vi "Spindle_load_RT_truncated (SubVI).vi"(9 "?":T1, 10 "concatenated string 4":string, 11 "String":string) -> (0 "error out":errorcluster, 1 "content 4":string, 2 "content1 2":string, 3 "output cluster":T1, 4 "empty? 2":bool, 5 "concatenated string":string, 6 "load":string, 7 "concatenated string 2":string)   [LabVIEW 2017]
uses:
  MT_connect_data.ctl
  <vilib>/regexp/Match Regular Expression.xnode
  <vilib>/addons/internet/NI_InternetTK_Core_VIs.lvlib
panel:
  out "Position A 2":string
  out "content 7":string
  out "content 6":string
  out "after match":string
  out "Z_position":string
  out "X_position":string
  out "Y_poistion":string
  out "concatenated string 6":string
  out "content 3":string
  out "Position B":string
  out "content 2":string
  out "concatenated string 5":string
  out "Position A":string
  out "Avail":string
  out "Tool_ID":string
  out "Program_name":string
  out "Controller_Mode":string
  out "Line_code":string
  out "program_status":string
  out "Block":string
  out "feeover":string
  out "Speedover":string
  out "path feedrate":string
  out "content":string
  out "error out 2":errorcluster
  out "spindle speed":string
  out "content 5":string
  out "empty? 3":bool
  out "after match 3":string
  out "content1 3":string
  out "concatenated string 3":string
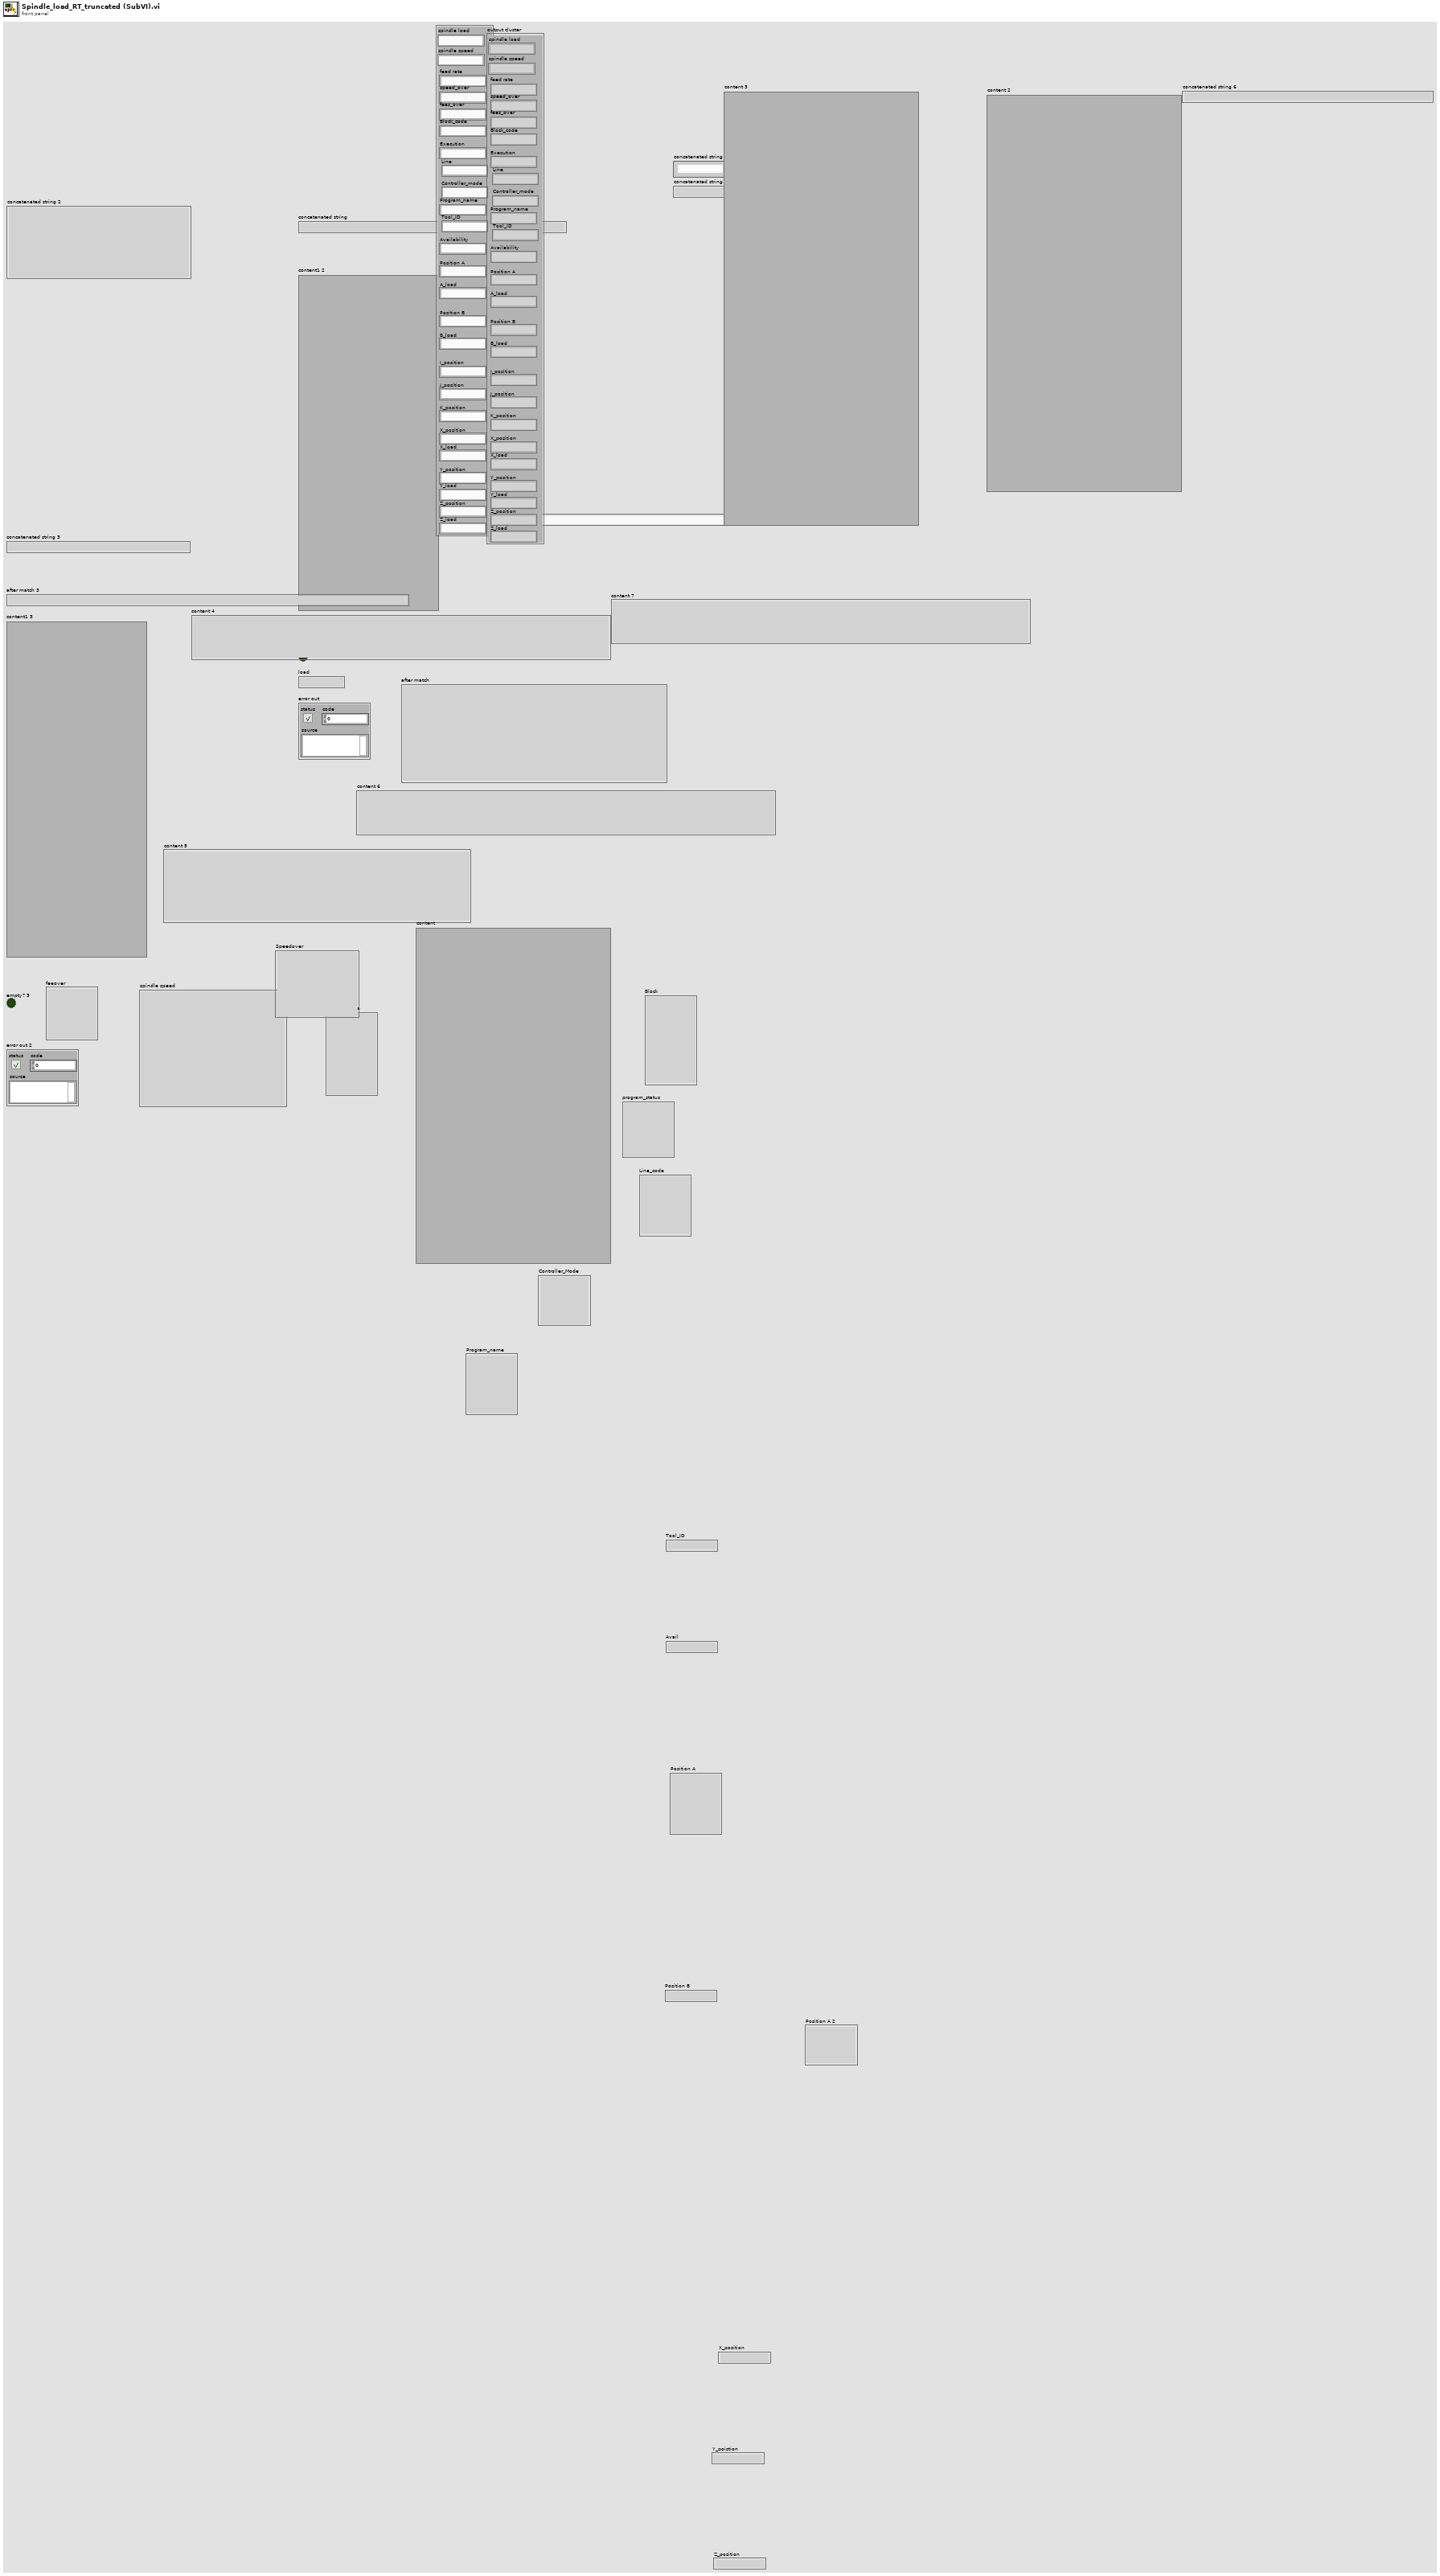
[diagram p1: front panel]
types:
  T1 = typedef "MT_connect_data.ctl" = cluster{"spindle load ":string, "spindle speed ":string, "feed rate":string, "speed_over":string, "fees_over":string, "Block_code":string, "Execution":string, "Line":string, "Controller_mode":string, "Program_name":string, "Tool_ID":string, "Availability":string, "Position A":string, "A_load":string, "Position B":string, "B_load":string, "I_position":string, "J_position":string, "K_position":string, "X_position":string, "X_load":string, "Y_position":string, "Y_load":string, "Z_position":string, "Z_load":string}
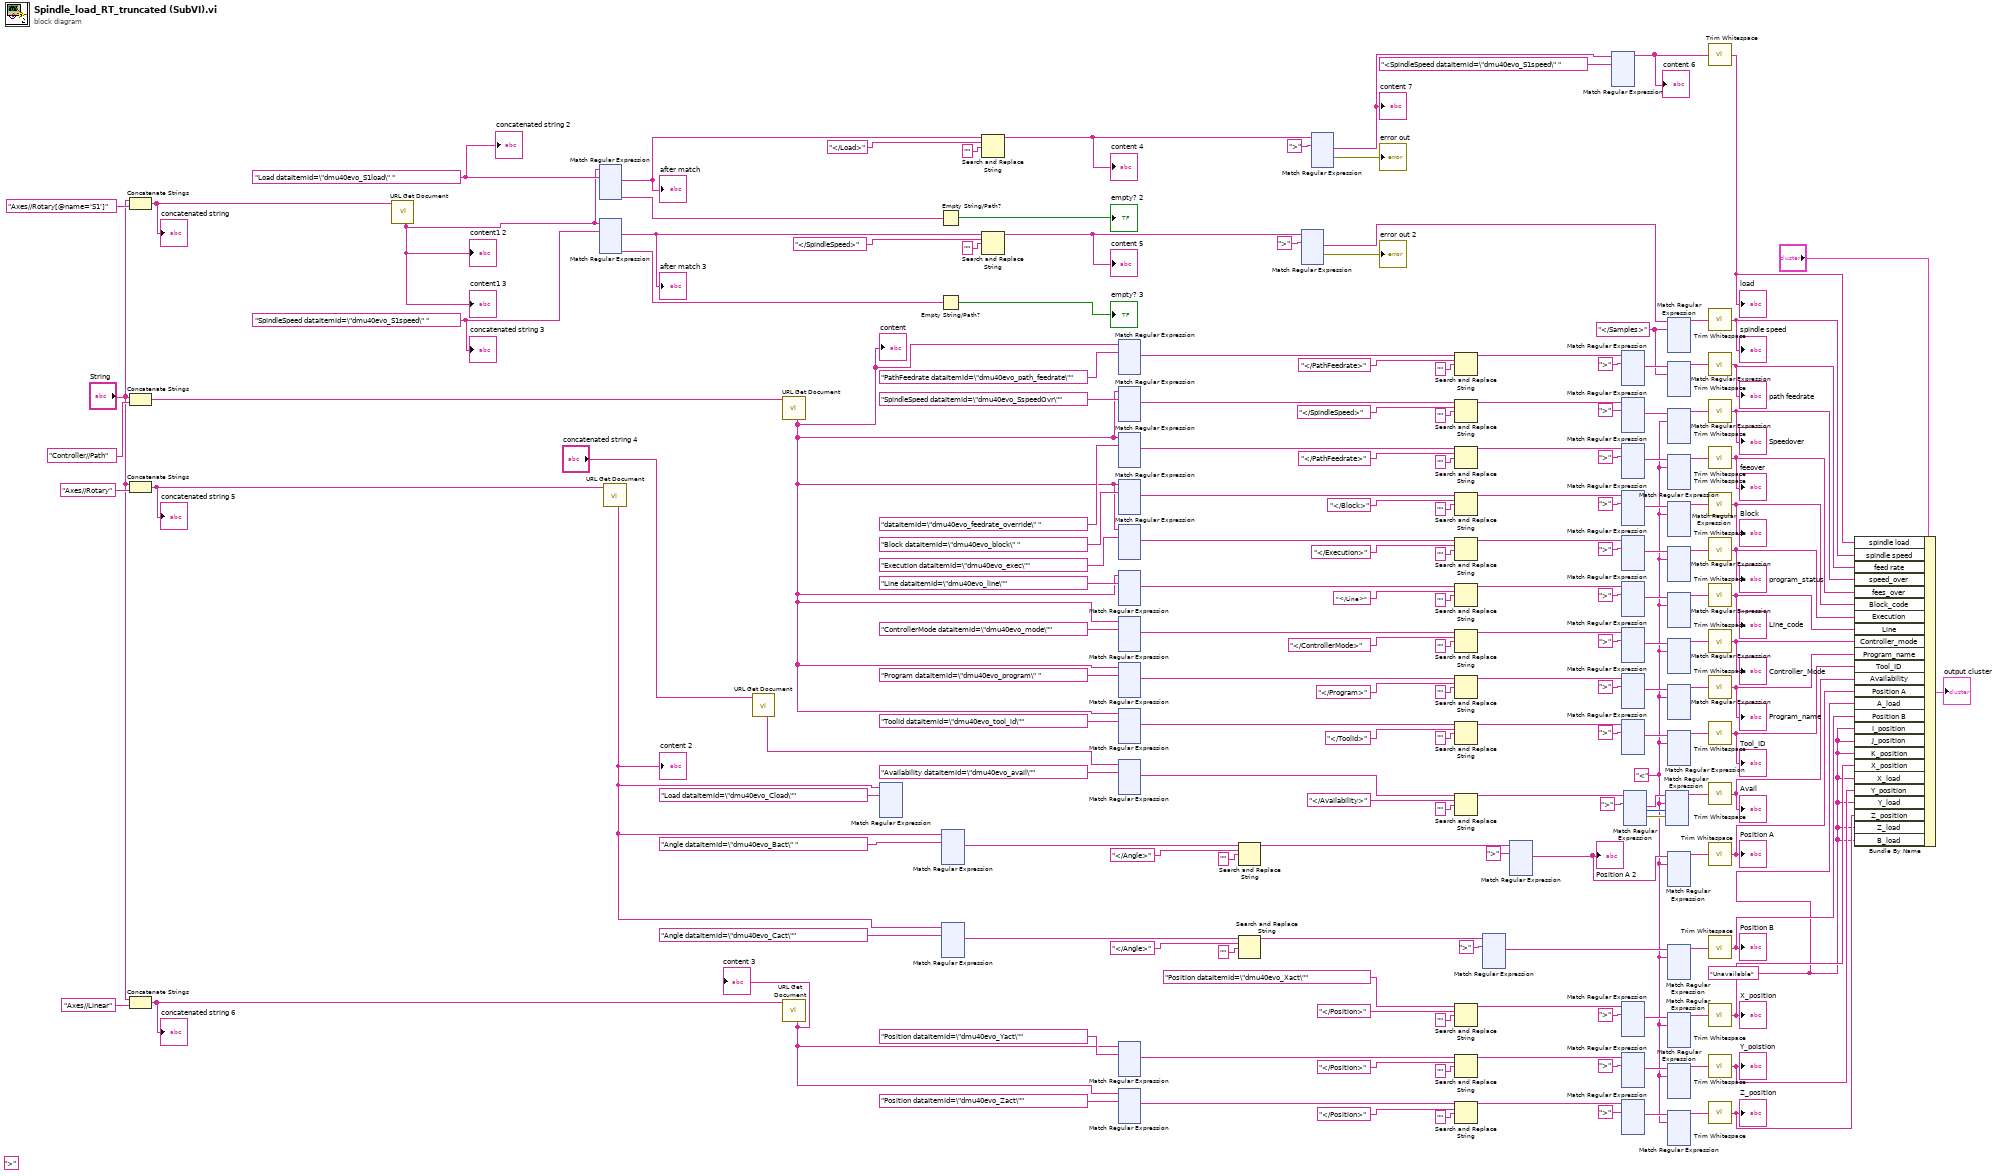
[diagram p0: block diagram]
diagram:
  w2 = "<" ("string")
  w1 = "Unavailable" ("I_position")
  w38 = "</Samples>" ("string")
  (unwired) ">" ("string")
  w170 = "SpindleSpeed dataItemId=\"dmu40evo_S1speed\" " ("regular expression")
  w181 = "Load dataItemId=\"dmu40evo_S1load\" " ("regular expression")
  n1 = Concatenate Strings("String", "Axes//Rotary[@name='S1']" ("string")) -> (w176:string)
  "concatenated string" <- w176
  n2 = Concatenate Strings("String", "Controller//Path" ("string")) -> (w157:string)
  n3 = Concatenate Strings("String", "Axes//Rotary" ("string")) -> (w67:string)
  "concatenated string 5" <- w67
  n4 = Concatenate Strings("String", "Axes//Linear" ("string")) -> (w66:string)
  "concatenated string 6" <- w66
  n5 = call <vilib>:"URL Get Document.vi"("URL"=w176) -> ("content"=w162:string)  [unwired: 6 in, 4 out]
  "content1 2" <- w162
  "content1 3" <- w162
  n6 = xnode "Match Regular Expression"("input string"=w162, "regular expression"=w181) -> ("after match"=w173:string, "submatch 1"=w175:string)  [unwired: 4 in, 4 out]
  "after match" <- w173
  n7 = xnode "Match Regular Expression"("input string"=w162, "regular expression"=w170) -> ("after match"=w164:string, "submatch 1"=w166:string)  [unwired: 4 in, 4 out]
  "after match 3" <- w164
  n8 = call <vilib>:"URL Get Document.vi"("URL"=w67) -> ("content"=w71:string)  [unwired: 6 in, 4 out]
  "content 2" <- w71
  n9 = call <vilib>:"URL Get Document.vi"("URL"="concatenated string 4") -> ("content"=w92:string)  [unwired: 6 in, 4 out]
  n10 = call <vilib>:"URL Get Document.vi"("URL"=w157) -> ("content"=w91:string)  [unwired: 6 in, 4 out]
  "content" <- w91
  n11 = call <vilib>:"URL Get Document.vi"("URL"=w66) -> ("content"=w48:string)  [unwired: 6 in, 4 out]
  "content 3" <- w48
  n12 = xnode "Match Regular Expression"("input string"=w71, "regular expression"="Load dataItemId=\"dmu40evo_Cload\"") -> ()  [unwired: 4 in, 6 out]
  n13 = Empty String/Path?(string/path=w175) -> (empty?=→"empty? 2":bool)
  n14 = Empty String/Path?(string/path=w166) -> (empty?=→"empty? 3":bool)
  n15 = xnode "Match Regular Expression"("input string"=w71, "regular expression"="Angle dataItemId=\"dmu40evo_Bact\" ") -> ("after match"=w84:string)  [unwired: 4 in, 5 out]
  n16 = xnode "Match Regular Expression"("input string"=w71, "regular expression"="Angle dataItemId=\"dmu40evo_Cact\"") -> ("after match"=w73:string)  [unwired: 4 in, 5 out]
  n17 = Search and Replace String(input string=w173, search string="</Load>" ("string"), replace string="" ("string")) -> (result string=w172:string)  [unwired: 5 in, 3 out]
  "content 4" <- w172
  n18 = Search and Replace String(input string=w164, search string="</SpindleSpeed>" ("string"), replace string="" ("string")) -> (result string=w163:string)  [unwired: 5 in, 3 out]
  "content 5" <- w163
  n19 = xnode "Match Regular Expression"("input string"=w91, "regular expression"="PathFeedrate dataItemId=\"dmu40evo_path_feedrate\"") -> ("after match"=w155:string)  [unwired: 4 in, 5 out]
  n20 = xnode "Match Regular Expression"("input string"=w91, "regular expression"="SpindleSpeed dataItemId=\"dmu40evo_SspeedOvr\"") -> ("after match"=w143:string)  [unwired: 4 in, 5 out]
  n21 = xnode "Match Regular Expression"("input string"=w91, "regular expression"="dataItemId=\"dmu40evo_feedrate_override\" ") -> ("after match"=w142:string)  [unwired: 4 in, 5 out]
  n22 = xnode "Match Regular Expression"("input string"=w91, "regular expression"="Block dataItemId=\"dmu40evo_block\" ") -> ("after match"=w129:string)  [unwired: 4 in, 5 out]
  n23 = xnode "Match Regular Expression"("input string"=w91, "regular expression"="Execution dataItemId=\"dmu40evo_exec\"") -> ("after match"=w121:string)  [unwired: 4 in, 5 out]
  n24 = xnode "Match Regular Expression"("input string"=w91, "regular expression"="Line dataItemId=\"dmu40evo_line\"") -> ("after match"=w120:string)  [unwired: 4 in, 5 out]
  n25 = xnode "Match Regular Expression"("input string"=w91, "regular expression"="ControllerMode dataItemId=\"dmu40evo_mode\"") -> ("after match"=w116:string)  [unwired: 4 in, 5 out]
  n26 = xnode "Match Regular Expression"("input string"=w91, "regular expression"="Program dataItemId=\"dmu40evo_program\" ") -> ("after match"=w107:string)  [unwired: 4 in, 5 out]
  n27 = xnode "Match Regular Expression"("input string"=w91, "regular expression"="ToolId dataItemId=\"dmu40evo_tool_id\"") -> ("after match"=w104:string)  [unwired: 4 in, 5 out]
  n28 = xnode "Match Regular Expression"("input string"=w92, "regular expression"="Availability dataItemId=\"dmu40evo_avail\"") -> ("after match"=w95:string)  [unwired: 4 in, 5 out]
  n29 = xnode "Match Regular Expression"("input string"=w48, "regular expression"="Position dataItemId=\"dmu40evo_Yact\"") -> ("after match"=w63:string)  [unwired: 4 in, 5 out]
  n30 = xnode "Match Regular Expression"("input string"=w48, "regular expression"="Position dataItemId=\"dmu40evo_Zact\"") -> ("after match"=w50:string)  [unwired: 4 in, 5 out]
  n31 = Search and Replace String(input string=w84, search string="</Angle>" ("string"), replace string="" ("string")) -> (result string=w85:string)  [unwired: 5 in, 3 out]
  n32 = Search and Replace String(input string=w73, search string="</Angle>" ("string"), replace string="" ("string")) -> (result string=w72:string)  [unwired: 5 in, 3 out]
  n33 = xnode "Match Regular Expression"("input string"=w163, "regular expression"=">" ("string")) -> ("after match"=w41:string, "error out"=→"error out 2":errorcluster)  [unwired: 4 in, 4 out]
  n34 = xnode "Match Regular Expression"("input string"=w172, "regular expression"=">" ("string")) -> ("after match"=w42:string, "error out"=→"error out":errorcluster)  [unwired: 4 in, 4 out]
  "content 7" <- w42
  n35 = Search and Replace String(input string=w155, search string="</PathFeedrate>" ("string"), replace string="" ("string")) -> (result string=w150:string)  [unwired: 5 in, 3 out]
  n36 = Search and Replace String(input string=w143, search string="</SpindleSpeed>" ("string"), replace string="" ("string")) -> (result string=w148:string)  [unwired: 5 in, 3 out]
  n37 = Search and Replace String(input string=w142, search string="</PathFeedrate>" ("string"), replace string="" ("string")) -> (result string=w137:string)  [unwired: 5 in, 3 out]
  n38 = Search and Replace String(input string=w129, search string="</Block>" ("string"), replace string="" ("string")) -> (result string=w134:string)  [unwired: 5 in, 3 out]
  n39 = Search and Replace String(input string=w121, search string="</Execution>" ("string"), replace string="" ("string")) -> (result string=w119:string)  [unwired: 5 in, 3 out]
  n40 = Search and Replace String(input string=w120, search string="</Line>" ("string"), replace string="" ("string")) -> (result string=w118:string)  [unwired: 5 in, 3 out]
  n41 = Search and Replace String(input string=w116, search string="</ControllerMode>" ("string"), replace string="" ("string")) -> (result string=w117:string)  [unwired: 5 in, 3 out]
  n42 = Search and Replace String(input string=w107, search string="</Program>" ("string"), replace string="" ("string")) -> (result string=w106:string)  [unwired: 5 in, 3 out]
  n43 = Search and Replace String(input string=w104, search string="</ToolId>" ("string"), replace string="" ("string")) -> (result string=w105:string)  [unwired: 5 in, 3 out]
  n44 = Search and Replace String(input string=w95, search string="</Availability>" ("string"), replace string="" ("string")) -> (result string=w94:string)  [unwired: 5 in, 3 out]
  n45 = Search and Replace String(input string="Position dataItemId=\"dmu40evo_Xact\"" ("regular expression"), search string="</Position>" ("string"), replace string="" ("string")) -> (result string=w58:string)  [unwired: 5 in, 3 out]
  n46 = Search and Replace String(input string=w63, search string="</Position>" ("string"), replace string="" ("string")) -> (result string=w64:string)  [unwired: 5 in, 3 out]
  n47 = Search and Replace String(input string=w50, search string="</Position>" ("string"), replace string="" ("string")) -> (result string=w49:string)  [unwired: 5 in, 3 out]
  n48 = xnode "Match Regular Expression"("input string"=w72, "regular expression"=">" ("string")) -> ("after match"=w20:string)  [unwired: 4 in, 5 out]
  n49 = xnode "Match Regular Expression"("input string"=w85, "regular expression"=">" ("string")) -> ("after match"=w16:string)  [unwired: 4 in, 5 out]
  "Position A 2" <- w16
  n50 = xnode "Match Regular Expression"("input string"=w42, "regular expression"="<SpindleSpeed dataItemId=\"dmu40evo_S1speed\" ") -> ("before match"=w43:string)  [unwired: 4 in, 5 out]
  "content 6" <- w43
  n51 = xnode "Match Regular Expression"("input string"=w150, "regular expression"=">" ("string")) -> ("after match"=w39:string)  [unwired: 4 in, 5 out]
  n52 = xnode "Match Regular Expression"("input string"=w148, "regular expression"=">" ("string")) -> ("after match"=w3:string)  [unwired: 4 in, 5 out]
  n53 = xnode "Match Regular Expression"("input string"=w137, "regular expression"=">" ("string")) -> ("after match"=w6:string)  [unwired: 4 in, 5 out]
  n54 = xnode "Match Regular Expression"("input string"=w134, "regular expression"=">" ("string")) -> ("after match"=w9:string)  [unwired: 4 in, 5 out]
  n55 = xnode "Match Regular Expression"("input string"=w119, "regular expression"=">" ("string")) -> ("after match"=w34:string)  [unwired: 4 in, 5 out]
  n56 = xnode "Match Regular Expression"("input string"=w118, "regular expression"=">" ("string")) -> ("after match"=w31:string)  [unwired: 4 in, 5 out]
  n57 = xnode "Match Regular Expression"("input string"=w117, "regular expression"=">" ("string")) -> ("after match"=w29:string)  [unwired: 4 in, 5 out]
  n58 = xnode "Match Regular Expression"("input string"=w106, "regular expression"=">" ("string")) -> ("after match"=w23:string)  [unwired: 4 in, 5 out]
  n59 = xnode "Match Regular Expression"("input string"=w105, "regular expression"=">" ("string")) -> ("after match"=w22:string)  [unwired: 4 in, 5 out]
  n60 = xnode "Match Regular Expression"("input string"=w58, "regular expression"=">" ("string")) -> ("after match"=w19:string)  [unwired: 4 in, 5 out]
  n61 = xnode "Match Regular Expression"("input string"=w64, "regular expression"=">" ("string")) -> ("after match"=w18:string)  [unwired: 4 in, 5 out]
  n62 = xnode "Match Regular Expression"("input string"=w49, "regular expression"=">" ("string")) -> ("after match"=w17:string)  [unwired: 4 in, 5 out]
  n63 = xnode "Match Regular Expression"("input string"=w94, "regular expression"=">" ("string")) -> ("after match"=w21:string, "offset past match"=w25:i32, "error out"=w24:errorcluster)  [unwired: 4 in, 3 out]
  n64 = xnode "Match Regular Expression"("input string"=w21, "regular expression"=w2, "offset (0)"=w25, "error in"=w24) -> ("before match"=w15:string)  [unwired: 2 in, 5 out]
  n65 = xnode "Match Regular Expression"("input string"=w41, "regular expression"=w38) -> ("before match"=w40:string)  [unwired: 4 in, 5 out]
  n66 = xnode "Match Regular Expression"("input string"=w39, "regular expression"=w38) -> ("before match"=w37:string)  [unwired: 4 in, 5 out]
  n67 = xnode "Match Regular Expression"("input string"=w3, "regular expression"=w2) -> ("before match"=w36:string)  [unwired: 4 in, 5 out]
  n68 = xnode "Match Regular Expression"("input string"=w6, "regular expression"=w2) -> ("before match"=w7:string)  [unwired: 4 in, 5 out]
  n69 = xnode "Match Regular Expression"("input string"=w9, "regular expression"=w2) -> ("before match"=w8:string)  [unwired: 4 in, 5 out]
  n70 = xnode "Match Regular Expression"("input string"=w34, "regular expression"=w2) -> ("before match"=w33:string)  [unwired: 4 in, 5 out]
  n71 = xnode "Match Regular Expression"("input string"=w31, "regular expression"=w2) -> ("before match"=w30:string)  [unwired: 4 in, 5 out]
  n72 = xnode "Match Regular Expression"("input string"=w29, "regular expression"=w2) -> ("before match"=w28:string)  [unwired: 4 in, 5 out]
  n73 = xnode "Match Regular Expression"("input string"=w23, "regular expression"=w2) -> ("before match"=w27:string)  [unwired: 4 in, 5 out]
  n74 = xnode "Match Regular Expression"("input string"=w22, "regular expression"=w2) -> ("before match"=w26:string)  [unwired: 4 in, 5 out]
  n75 = xnode "Match Regular Expression"("input string"=w16, "regular expression"=w2) -> ("before match"=w14:string)  [unwired: 4 in, 5 out]
  n76 = xnode "Match Regular Expression"("input string"=w20, "regular expression"=w2) -> ("before match"=w13:string)  [unwired: 4 in, 5 out]
  n77 = xnode "Match Regular Expression"("input string"=w19, "regular expression"=w2) -> ("before match"=w12:string)  [unwired: 4 in, 5 out]
  n78 = xnode "Match Regular Expression"("input string"=w18, "regular expression"=w2) -> ("before match"=w11:string)  [unwired: 4 in, 5 out]
  n79 = xnode "Match Regular Expression"("input string"=w17, "regular expression"=w2) -> ("before match"=w10:string)  [unwired: 4 in, 5 out]
  n80 = call <vilib>:"Trim Whitespace.vi"("string"=w43) -> ("trimmed string"=w160:string)  [unwired: 1 in]
  "load" <- w160
  n81 = call <vilib>:"Trim Whitespace.vi"("string"=w40) -> ("trimmed string"=w159:string)  [unwired: 1 in]
  "spindle speed" <- w159
  n82 = call <vilib>:"Trim Whitespace.vi"("string"=w37) -> ("trimmed string"=w149:string)  [unwired: 1 in]
  "path feedrate" <- w149
  n83 = call <vilib>:"Trim Whitespace.vi"("string"=w36) -> ("trimmed string"=w136:string)  [unwired: 1 in]
  "Speedover" <- w136
  n84 = call <vilib>:"Trim Whitespace.vi"("string"=w7) -> ("trimmed string"=w135:string)  [unwired: 1 in]
  "feeover" <- w135
  n85 = call <vilib>:"Trim Whitespace.vi"("string"=w8) -> ("trimmed string"=w5:string)  [unwired: 1 in]
  "Block" <- w5
  n86 = call <vilib>:"Trim Whitespace.vi"("string"=w33) -> ("trimmed string"=w90:string)  [unwired: 1 in]
  "program_status" <- w90
  n87 = call <vilib>:"Trim Whitespace.vi"("string"=w30) -> ("trimmed string"=w32:string)  [unwired: 1 in]
  "Line_code" <- w32
  n88 = call <vilib>:"Trim Whitespace.vi"("string"=w28) -> ("trimmed string"=w89:string)  [unwired: 1 in]
  "Controller_Mode" <- w89
  n89 = call <vilib>:"Trim Whitespace.vi"("string"=w27) -> ("trimmed string"=w88:string)  [unwired: 1 in]
  "Program_name" <- w88
  n90 = call <vilib>:"Trim Whitespace.vi"("string"=w26) -> ("trimmed string"=w87:string)  [unwired: 1 in]
  "Tool_ID" <- w87
  n91 = call <vilib>:"Trim Whitespace.vi"("string"=w15) -> ("trimmed string"=w86:string)  [unwired: 1 in]
  "Avail" <- w86
  n92 = call <vilib>:"Trim Whitespace.vi"("string"=w14) -> ("trimmed string"=w70:string)  [unwired: 1 in]
  "Position A" <- w70
  n93 = call <vilib>:"Trim Whitespace.vi"("string"=w13) -> ("trimmed string"=w69:string)  [unwired: 1 in]
  "Position B" <- w69
  n94 = call <vilib>:"Trim Whitespace.vi"("string"=w12) -> ("trimmed string"=w47:string)  [unwired: 1 in]
  "X_position" <- w47
  n95 = call <vilib>:"Trim Whitespace.vi"("string"=w11) -> ("trimmed string"=w46:string)  [unwired: 1 in]
  "Y_poistion" <- w46
  n96 = call <vilib>:"Trim Whitespace.vi"("string"=w10) -> ("trimmed string"=w45:string)  [unwired: 1 in]
  "Z_position" <- w45
  n97 = Bundle By Name(cluster="?", "spindle load"=w160, "spindle speed"=w159, "feed rate"=w149, "speed_over"=w136, "fees_over"=w135, "Block_code"=w5, "Execution"=w90, "Line"=w32, "Controller_mode"=w89, "Program_name"=w88, "Tool_ID"=w87, "Availability"=w86, "Position A"=w70, "A_load"=w1, "Position B"=w69, "I_position"=w1, "J_position"=w1, "K_position"=w1, "X_position"=w47, "X_load"=w1, "Y_position"=w46, "Y_load"=w1, "Z_position"=w45, "Z_load"=w1, "B_load"=w1) -> (→"output cluster":T1)
  "concatenated string 2" <- w181
  "concatenated string 3" <- w170
